vi "ATMonochromator_monitorCommand_updateMonochromatorSetup.vi"(8 "error in (no error)":errorcluster, 11 "command_updateMonochromatorSetup_Ctl":T1) -> (0 "error out":errorcluster, 2 "function return":i32, 3 "command_updateMonochromatorSetup_Ctl out":T1)   [LabVIEW 2016, in "SALLV_ATMonochromator.lvlib"]
doc: "int ATMonochromator_shm_monitorCommand_updateMonochromatorSetupLV(ATMonochromator_command_updateMonochromatorSetupLV *command_updateMonochromatorSetup_Ctl );"
uses:
  SALLV_ATMonochromator.lvlib
  DataTypes/command_updateMonochromatorSetup.ctl
  SALLV_ATMonochromator.so
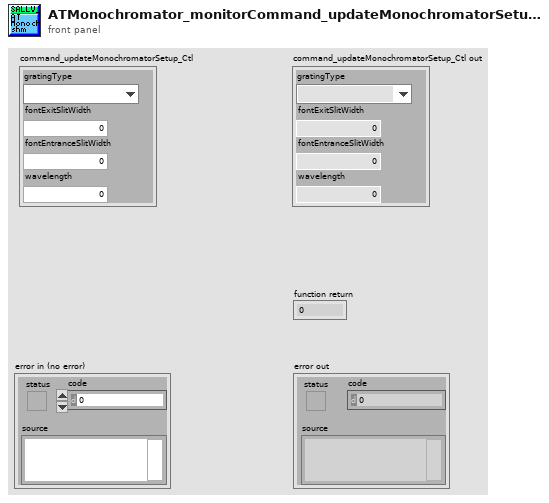
[diagram p1: front panel]
types:
  T1 = typedef "SALLV_ATMonochromator.lvlib/command_updateMonochromatorSetup.ctl" = cluster{"gratingType":enum32{"", "Blue", "Red", "Mirror"}, "fontExitSlitWidth":dbl, "fontEntranceSlitWidth":dbl, "wavelength":dbl}
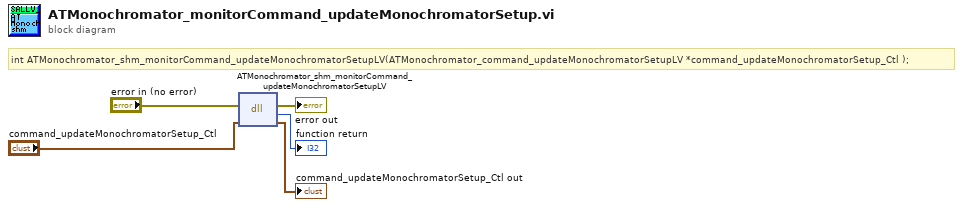
[diagram p0: block diagram]
diagram:
  # "int ATMonochromator_shm_monitorCommand_updateMonochromatorSetupLV(ATMonochromator_command_updateMonochromatorSetupLV *command_updateMonochromatorSetup_Ctl );"
  n1 = dll-call lib="home/harini/tcs/SALLV_ATMonochromator/SALLV_ATMonochromator.*" fn="ATMonochromator_shm_monitorCommand_updateMonochromatorSetupLV"(error in="error in (no error)", "command_updateMonochromatorSetup_Ctl"="command_updateMonochromatorSetup_Ctl") -> (error out=→"error out":errorcluster, →"function return":i32, "command_updateMonochromatorSetup_Ctl"=→"command_updateMonochromatorSetup_Ctl out":T1)  [unwired: 2 in, 1 out]
